vi "ABR3 Main Panel.vi"(11 "State (in)":T11) -> (3 "State":T11)   [LabVIEW 2020]
uses:
  epl-vi-lib/Utility VIs/Buttons/KCheckmarkBoolean 2.ctl
  epl-vi-lib/Utility VIs/Type Defs/Left-Right ring.ctl
  epl-vi-lib/Signal Synthesis VIs/Controls/Advanced Filter XCtl/Advanced Filter XCtl.xctl
  CFTS Main Panel SubVIs/CFTS-Experiment State.ctl
  TypeDefs/ABR3-Analysis State.ctl
  Threshold Estimation VIs/ABR3-Threshold Estimation Result.ctl
  TypeDefs/ABR3-Masker Spec.ctl
  epl-vi-lib/Signal Synthesis VIs/Controls/Level XCtl/Level XCtl.xctl
  TypeDefs/ABR3-Parameters.ctl
  TypeDefs/ABR3-Stimulus.ctl
  TypeDefs/ABR-Waveform Enum.ctl
  epl-vi-lib/Signal Synthesis VIs/Filter VIs/Filter-Bandwidth Units.ctl
  epl-vi-lib/Signal Synthesis VIs/Controls/Level XCtl/Level Units.ctl
  TypeDefs/ABR3-Sequence Spec.ctl
  TypeDefs/ABR3-Controls.ctl
  TypeDefs/ABR3-Response.ctl
  TypeDefs/ABR3-Hidden Params.ctl
  Threshold Estimation VIs/ABR3-Threshold Estimation Parameters.ctl
  <vilib>/Utility/sysdir.llb/System Directory Type.ctl
panel:
  out "Thr":string caption="Threshold (dB SPL)"
  out "User":string
  out "Run #":u16
  out "ID #":u16
  in  "Presets":u16(ring) items=["bpn", "memr chirp", "signal only", "test controls", "test", "with masker", "--- defaults ---"]
  out "resume signal":bool
  out "Masker state":bool
  in  "Last user":string
  out "exit signal":bool
  in  "Tab Control":enum32{"Stimulus", "Masker"}(tab)=enum."Masker"
  in  "Stimulus":T3={"Ear"=enum."Left", "Waveform"=enum."FILE", "Frequency (kHz)"="", "Rep rate (/sec)"=80.0, "Alternate Polarity"=FALSE, "Filenames"="", "Level (dB SPL)"=30.0, "Folder"=path "", "Chirp"={"Type"=enum."AN latency-corrected", "Duration (ms)"=30.0, "Fmin (kHz)"=30.0, "Fmax (kHz)"=80.0, "Precompensate"=FALSE}, "Noise"={"Seed"=0.0, "InvFilt"=FALSE, "Audiogram Comp"=FALSE, "Audiogram File"=path "", "Filter"={"Type"=enum."Lowpass", "CF (kHz)"=0.0, "BW (kHz)"=0.0, "Cascade"=FALSE, "Quadrature"=FALSE, "Scale Factor"=0.0, "Stages"=[], "Class"=enum."Elliptic", "Order"=0, "BWUnits"=enum."Linear"}}}
  in  "File browse":bool
  in  "Masker":T4
  out "Running":bool
  out "Abort":bool
  in  "Controls":T6
  in  "Sequence":T7={"Start (dB)"=20, "Stop (dB)"=80, "Step (dB)"=5, "Var"=enum."Signal", "Order"=enum."Sequential"} {"Start (dB)" step=5}
  in  "Response":T8={"Gain"=10000, "Averages"=512, "Window (ms)"=8.5, "Thr Fast Steps"=1.5, "AI Fs"=25000.0} {"Thr Fast Steps" format="%.2f"; "Window (ms)" format="%.2f"}
  in  "CAP or ABR":enum16{"CAP", "ABR"}(ring)=enum."ABR" caption="Measure what"
  out "CM":cluster{dbl[], dbl[]}[](graph) caption="\"CM\""
  out "Neural":cluster{dbl[], dbl[]}[](graph)
  out "load params":bool
  out "redisplay":bool
  out "settings":path
  in  "finished":errorcluster
  out "Wave 1":cluster{dbl[], dbl[]}[](graph)
  out "Analysis":T9
  out "kHz":dbl=35.0
  out "MAX SPL":dbl=113.05999755859375 format="%.2f"
  out "SPL":dbl=35.0
  out "DataPath":path
  in  "Normalize traces":T12=TRUE caption="Normalize individual traces"
  in  "Start":bool
  in  "Exit":bool
  in  "Stop":bool
  out "I-O":cluster{dbl[], dbl[]}[](graph)
  in  "NOTES":string
  # "Level"
  # "Controls"
  # "Running Average"
  # "Response"
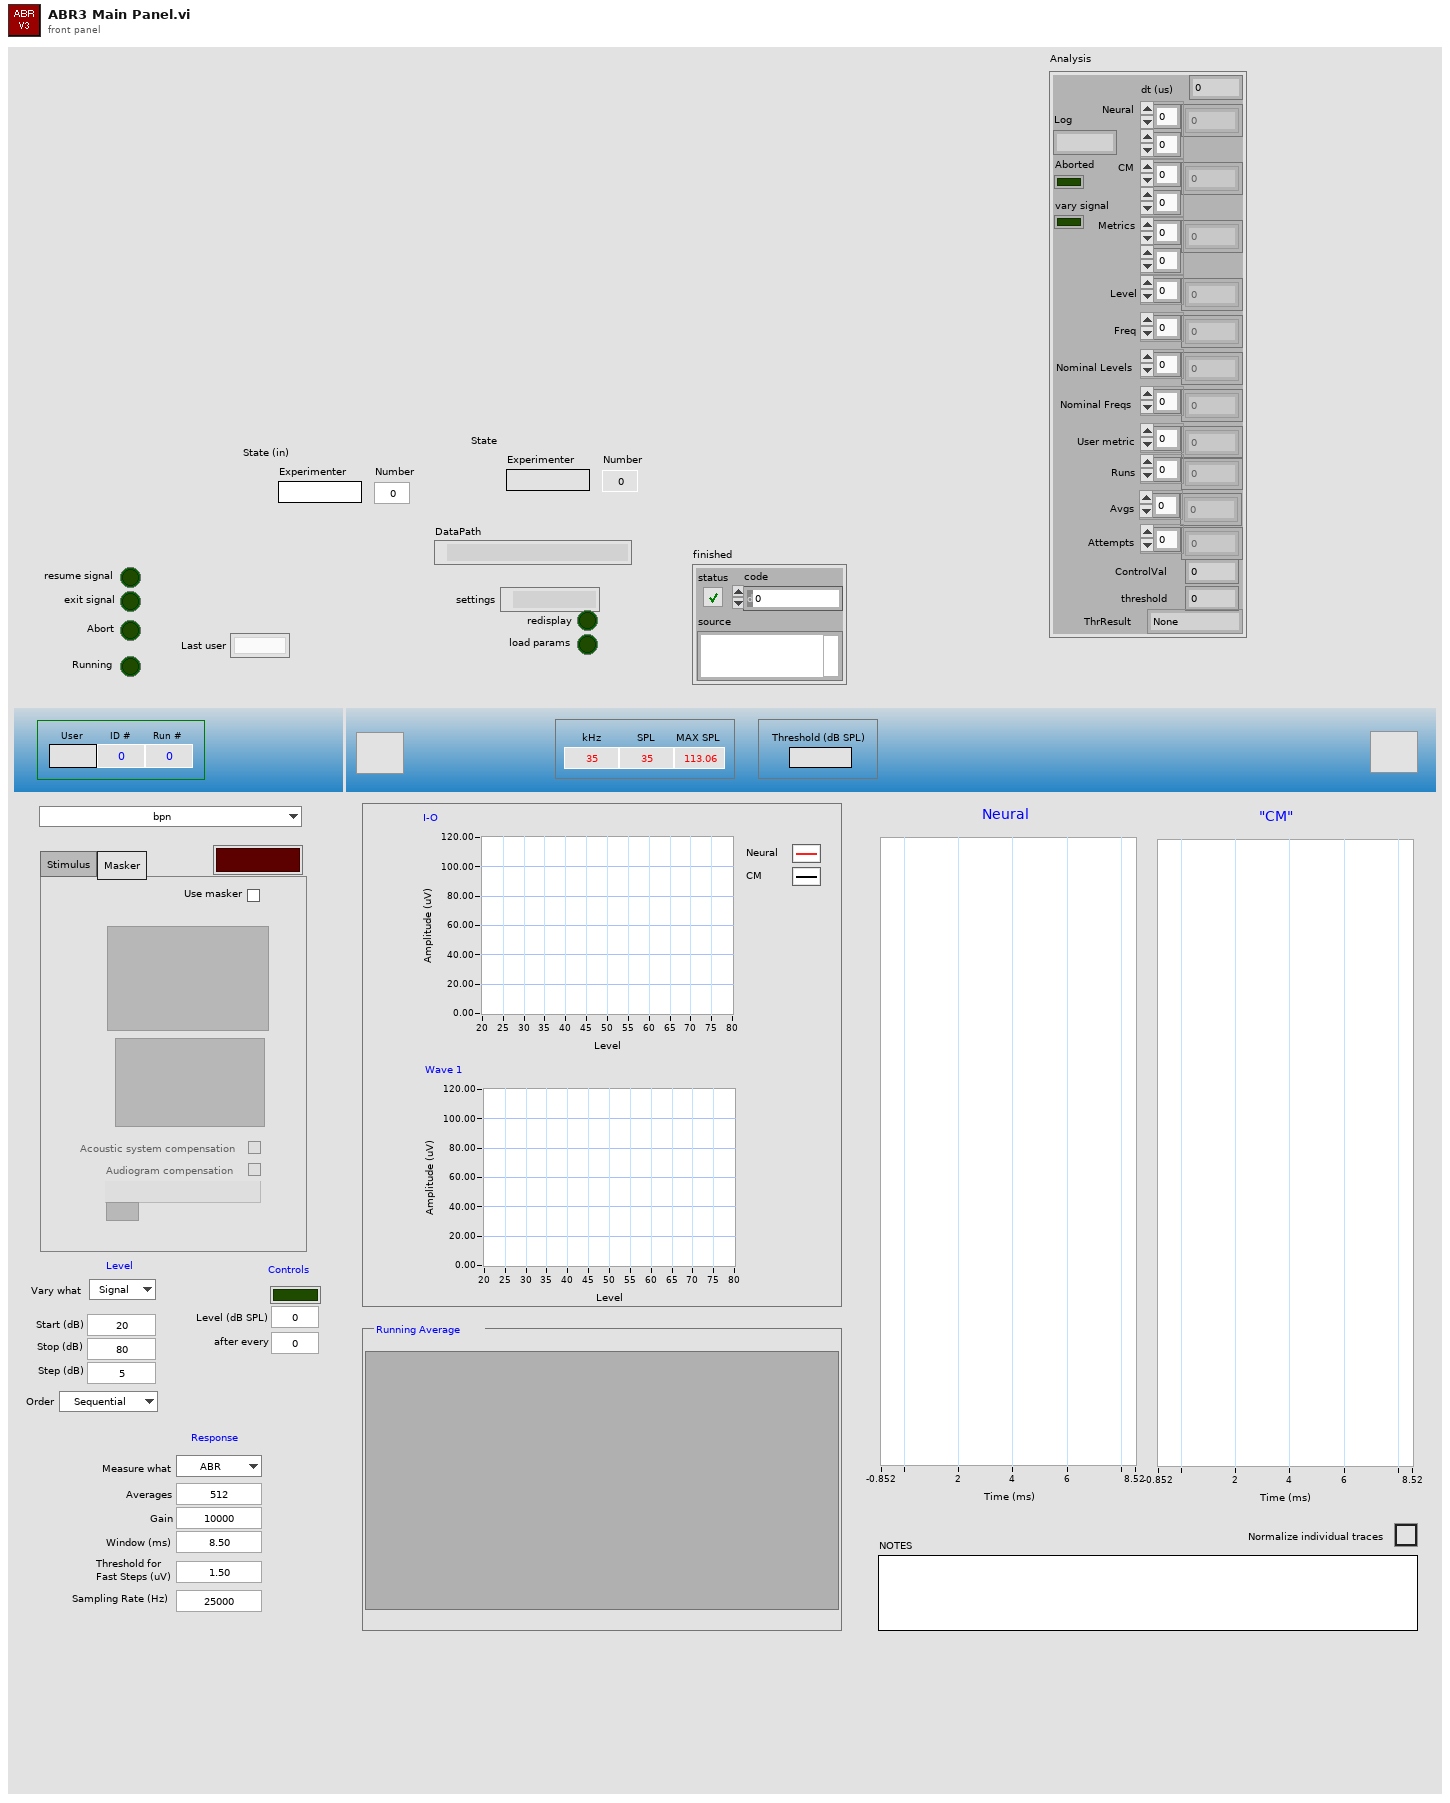
[diagram p1: front panel]
types:
  T1 = typedef "Left-Right ring.ctl" = enum16{"Right", "Left"}
  T2 = typedef "Filter-Bandwidth Units.ctl" = enum16{"Linear", "Octaves", "Min-Max"}
  T3 = cluster{"Ear":T1, "Waveform":enum16{"TONE PIP", "CLICK", "FILE", "CHIRP", "NOISE"}, "Frequency (kHz)":string, "Rep rate (/sec)":dbl, "Alternate Polarity":bool, "Filenames":string, "Level (dB SPL)":dbl, "Folder":path, "Chirp":cluster{"Type":enum16{"AN latency-corrected", "Arbitrary"}, "Duration (ms)":dbl, "Fmin (kHz)":dbl, "Fmax (kHz)":dbl, "Precompensate":bool}, "Noise":cluster{"Seed":dbl, "InvFilt":bool, "Audiogram Comp":bool, "Audiogram File":path, "Filter":cluster{"Type":enum16{"Lowpass", "Highpass", "Bandpass", "Bandstop", "OFF"}, "CF (kHz)":dbl, "BW (kHz)":dbl, "Cascade":bool, "Quadrature":bool, "Scale Factor":dbl, "Stages":cluster{"IIR Filter":cluster{"filter structure":enum32{"IIR 2nd Order", "IIR 4th Order"}, "Reverse Coefficients":dbl[], "Forward Coefficients":dbl[]}, "State":dbl[]}[], "Class":enum16{"Elliptic", "Butterworth"}, "Order":i32, "BWUnits":T2}}}
  T4 = typedef "ABR3-Masker Spec.ctl" = cluster{"Filter":cluster{"Type":enum16{"Lowpass", "Highpass", "Bandpass", "Bandstop", "OFF"}, "CF (kHz)":dbl, "BW (kHz)":dbl, "Cascade":bool, "Quadrature":bool, "Scale Factor":dbl, "Stages":cluster{"IIR Filter":cluster{"filter structure":enum32{"IIR 2nd Order", "IIR 4th Order"}, "Reverse Coefficients":dbl[], "Forward Coefficients":dbl[]}, "State":dbl[]}[], "Class":enum16{"Elliptic", "Butterworth"}, "Order":i32, "BWUnits":T2}, "Use masker":bool, "Level":cluster{"Level":dbl, "Units":T5, "Max":dbl, "Multiplier":dbl, "Cal File":path, "Cal":cluster{"Freq (Hz)":dbl[], "Mag (dB SPL)":dbl[], "Phase (deg)":dbl[]}}, "Audiogram Comp":bool, "Audiogram File":path, "InvFilt":bool}
  T5 = typedef "Level Units.ctl" = enum16{"dB atten", "dB SPL", "dB re 1 Vrms", "dB V/Hz½", "mW", "dB HL", "Volts", "dB mW"}
  T6 = cluster{"on":bool, "Dur (ms)":dbl, "spacing":i32}
  T7 = cluster{"Start (dB)":i32, "Stop (dB)":i32, "Step (dB)":i32, "Var":enum16{"Signal", "Masker"}, "Order":enum16{"Sequential", "Random"}}
  T8 = cluster{"Gain":i32, "Averages":i32, "Window (ms)":sgl, "Thr Fast Steps":sgl, "AI Fs":dbl}
  T9 = typedef "ABR3-Analysis State.ctl" = cluster{"dt (us)":dbl, "Neural":dbl[][], "CM":dbl[][], "Metrics":dbl[][], "Level":dbl[], "Freq":dbl[], "Nominal Levels":dbl[], "Nominal Freqs":dbl[], "User metric":dbl[], "Runs":i32[], "Avgs":i32[], "Attempts":i32[], "Log":string, "Aborted":bool, "ControlVal":dbl, "threshold":dbl, "vary signal":bool, "ThrResult":T10}
  T10 = typedef "ABR3-Threshold Estimation Result.ctl" = enum16{"None", "Power", "Sigmoid", "Power (noisy)", "Suprathreshold", "Invalid"}
  T11 = typedef "CFTS-Experiment State.ctl" = cluster{"Experimenter":string, "Number":u32, "Right":string, "Left":string, "Data Folder":path, "State File":path, "Version Info":string, "End Exposure Time":dbl, "Exposure Duration":string, "Run #":cluster{"CAP":i16, "ABR":i16, "DP":i16, "VsEP":i16, "MeasSeq":i16, "SubSeq":i16, "SFOAE":i16}}
  T12 = typedef "KCheckmarkBoolean 2.ctl" = bool
  T13 = typedef "ABR3-Threshold Estimation Parameters.ctl" = cluster{"Tmin (ms)":dbl, "Tmax (ms)":dbl, "CC criterion":dbl, "adjR2 criterion":dbl}
  T14 = typedef "ABR3-Parameters.ctl" = cluster{"CAP or ABR":enum16{"CAP", "ABR"}, "Stimulus":T15, "Masker":T4, "Sequence":T17, "Controls":T18, "Response":T19, "Hidden":T20}
  T15 = typedef "ABR3-Stimulus.ctl" = cluster{"Ear":T1, "Waveform":T16, "Frequency (kHz)":string, "Rep rate (/sec)":dbl, "Alternate Polarity":bool, "WavFiles":string, "Level (dB SPL)":dbl, "WavFolder":path, "Chirp":cluster{"Type":enum16{"AN latency-corrected", "Arbitrary"}, "Duration (ms)":dbl, "Fmin (kHz)":dbl, "Fmax (kHz)":dbl, "precompensate":bool}, "Noise":cluster{"Seed":i32, "InvFilt":bool, "AWeight":bool, "afile":path, "Filter":cluster{"Type":enum16{"Lowpass", "Highpass", "Bandpass", "Bandstop", "OFF"}, "CF (kHz)":dbl, "BW (kHz)":dbl, "Cascade":bool, "Quadrature":bool, "Scale Factor":dbl, "Stages":cluster{"IIR Filter":cluster{"filter structure":enum32{"IIR 2nd Order", "IIR 4th Order"}, "Reverse Coefficients":dbl[], "Forward Coefficients":dbl[]}, "State":dbl[]}[], "Class":enum16{"Elliptic", "Butterworth"}, "Order":i32, "BWUnits":T2}}}
  T16 = typedef "ABR-Waveform Enum.ctl" = enum16{"TONE PIP", "CLICK", "FILE", "CHIRP", "NOISE", "VERHULST"}
  T17 = typedef "ABR3-Sequence Spec.ctl" = cluster{"Start (dB)":i32, "Stop (dB)":i32, "Step (dB)":i32, "Var":enum16{"Signal", "Masker"}, "Order":enum16{"Sequential", "Random"}}
  T18 = typedef "ABR3-Controls.ctl" = cluster{"on":bool, "value":dbl, "spacing":i32}
  T19 = typedef "ABR3-Response.ctl" = cluster{"Gain":i32, "Averages":i32, "Window (ms)":sgl, "Thr Fast Steps":sgl, "AI Fs":dbl}
  T20 = typedef "ABR3-Hidden Params.ctl" = cluster{"AO Samp Rate Hz":dbl, "Duration (ms)":dbl, "Ramp (ms)":dbl, "Click width (us)":dbl}
  T21 = cluster{"Params":T14, "Threshold Estimation":T13}
  T22 = cluster{"I-O":refnum<vi>, "Neural":refnum<vi>, "CM":refnum<vi>, "Wave 1":refnum<vi>}
  T23 = typedef "ABR3-Runtime Data.ctl" = cluster{"Ceiling":dbl, "Threshold":dbl, "Crossed?":bool, "Step":i32, "Stop":i32, "Avgs":i32, "Level":dbl, "AI Npts":i32, "Doubled?":bool, "Gain":dbl, "NWindowPts":i32, "dt":dbl, "Cal":path, "Freq":dbl, "AO Channels":i32[], "AltPol":bool, "AO Npts":i32, "AO Fs":dbl, "Start":i32, "Stop max":i32, "Ear":T1, "Waveform":T16, "RepRate":dbl, "CAP or ABR":u16, "LMasker":dbl, "SeqVar":T24, "Reps/buffer":i32, "Avg Mode":enum16{"Neural/CM", "ANOW"}, "Wav":path, "Order":enum16{"Sequential", "Random"}, "Levels":dbl[], "ControlVal":dbl, "innerIndex":i32, "indexStep":i32}
  T24 = typedef "ABR3-Seq Var Enum.ctl" = enum16{"Signal Level", "Masker Level"}
  T25 = typedef "Stimulus Channel (Full).xctl/Full Stimulus Channel Data.ctl" = cluster{"Waveform":T26, "Filter":T43, "Burst":T44, "Level":T45, "Name":string, "Advanced":T46, "SAM":T47}
  T26 = typedef "Waveform XCtl.xctl/Waveform Data.ctl" = cluster{"Type":T27, "Tone":T28, "Pulse Train":T29, "Noise":T32, "File":T33, "FMSweep":T34, "Chirp Train":T35, "Complex Tone":cluster{"Params":T37, "Data":T39}, "Moving Ripple":T40}
  T27 = typedef "Waveform Enum.ctl" = enum16{"OFF", "Tone", "Noise", "Pulse Train", "File", "FM Sweep", "Chirp Train", "Complex Tone", "FM Tone", "Moving Ripple"}
  T28 = typedef "Tone Params.ctl" = cluster{"Frequency (kHz)":dbl, "Last Freq":dbl, "Last Phase":dbl}
  T29 = typedef "Pulse Train Params.ctl" = cluster{"Pulse width (us)":dbl, "Pulse rate (Hz)":dbl, "Gap (ms)":dbl, "Polarity":T30, "PT State":T31, "Asynch":bool}
  T30 = typedef "Pulse Polarity.ctl" = enum16{"POS", "NEG", "POS-NEG", "NEG-POS"}
  T31 = typedef "PT-Continuous State.ctl" = cluster{"Template":dbl[], "Nperiod":i32, "Index":i32, "Pulse Rate (Hz)":dbl, "Phase (cycles)":dbl, "Noff":i32}
  T32 = typedef "Noise Params.ctl" = cluster{"InvFilt":bool, "Noise":dbl[], "CurPt":i32, "Aweight":bool, "Seed":i32, "afile":path}
  T33 = typedef "StimFile-Params.ctl" = cluster{"Filename":path, "Signal":dbl[], "Channel":i32, "stream":bool, "offset":i32, "nreps":i32, "loops":i32, "Randomize":bool, "order":i32[], "Seed":i32, "Tokens":i32}
  T34 = typedef "FM Sweep Params.ctl" = cluster{"Rate (oct/s)":dbl, "Fmin (Hz)":dbl, "Fmax (Hz)":dbl, "Ramp (ms)":dbl, "Linear":bool}
  T35 = typedef "Chirp Train.ctl" = cluster{"Params":T36, "Data":cluster{"WF":dbl[]}}
  T36 = typedef "Chirp Train Params.ctl" = cluster{"Fmin (kHz)":dbl, "Fmax (kHz)":dbl, "Compensate":bool, "Duration (ms)":dbl}
  T37 = typedef "CT-Params.ctl" = cluster{"F0 (Hz)":dbl, "Band":cluster{"Flow (Hz)":dbl, "Fhigh (Hz)":dbl}, "Phase":T38, "Min F0 (Hz)":dbl, "Max F0 (Hz)":dbl, "ContinRandPhase":bool, "Max peak factor":dbl, "Max mod depth":dbl, "MinHarmNum":i32, "MaxHarmNum":i32, "Level Mode":enum16{"per component", "overall rms"}, "% jitter":dbl}
  T38 = typedef "CT-Phase Enum.ctl" = enum16{"Cosine", "Random", "Alternating"}
  T39 = typedef "CT-Runtime Data.ctl" = cluster{"Ncomp":i32, "MinHarm":i32, "Phase":dbl[], "Amplitude":dbl[], "Npts/frame":i32, "Last F0":dbl, "Fmin":dbl, "Fmax":dbl, "Lslope":dbl, "randphase":bool, "overall rms":bool, "fmult":dbl[], "jittered":bool}
  T40 = typedef "Moving Ripple.ctl" = cluster{"Params":T41, "Data":T42}
  T41 = typedef "Moving Ripple.Params.ctl" = cluster{"Fmin":dbl, "Fmax":dbl, "Density":dbl, "Velocity":dbl, "Depth":dbl, "Phase":dbl, "Comp/oct":i32}
  T42 = typedef "Moving Ripple.Data.ctl" = cluster{"Freq":dbl[], "A":dbl[], "phase":dbl[], "Phase":dbl}
  T43 = typedef "Advanced Filter XCtl.xctl/Filter Data.ctl" = cluster{"Type":enum16{"Lowpass", "Highpass", "Bandpass", "Bandstop", "OFF"}, "CF (kHz)":dbl, "BW (kHz)":dbl, "Cascade":bool, "Quadrature":bool, "Scale Factor":dbl, "Stages":cluster{"IIR Filter":cluster{"filter structure":enum32{"IIR 2nd Order", "IIR 4th Order"}, "Reverse Coefficients":dbl[], "Forward Coefficients":dbl[]}, "State":dbl[]}[], "Class":enum16{"Elliptic", "Butterworth"}, "Order":i32, "BWUnits":T2}
  T44 = typedef "Burst Control.xctl/Burst Data.ctl" = cluster{"Active":bool, "Delay (ms)":dbl, "Duration (ms)":dbl, "Ramp (ms)":dbl, "Rate (Hz)":dbl, "Trepeat (ms)":dbl, "Repeat":bool}
  T45 = typedef "Level XCtl.xctl/Level Data.ctl" = cluster{"Level":dbl, "Units":T5, "Max":dbl, "Multiplier":dbl, "Cal File":path, "Cal":cluster{"Freq (Hz)":dbl[], "Mag (dB SPL)":dbl[], "Phase (deg)":dbl[]}}
  T46 = typedef "Advanced Stimulus Options.xctl/Advanced Stimulus Options.ctl" = cluster{"Rep Mask":string, "AltPol":bool, "Var":string, "Expr":string, "Persist":bool}
  T47 = typedef "SAM Params.ctl" = cluster{"Active":bool, "Frequency (Hz)":dbl, "Depth":dbl, "Init Phase (cycles)":dbl, "phase (degrees)":dbl, "Asynch":bool}
  T48 = typedef "Multichannel (Full).xctl/Data.ctl" = T25[]
  T49 = enum8{"Enabled", "Disabled", "Disabled and Grayed Out"}
  T50 = cluster{"Shift":bool, "Ctrl":bool, "Alt":bool, "Cmd":bool, "Opt":bool}
  T51 = typedef "ABR3-Threshold Estimation Work.ctl" = cluster{"Threshold":dbl, "Criterion":dbl, "graphs":cluster{"X":dbl[], "Y":dbl[]}[], "Power2":string, "Sigmoid":string, "Result":T10}
  T52 = enum16{"TONE PIP", "CLICK", "FILE", "CHIRP", "NOISE"}
  T53 = cluster{"Params":T14, "Threshold Estimation Out":T13}
  T54 = typedef "System Directory Type.ctl" = i32
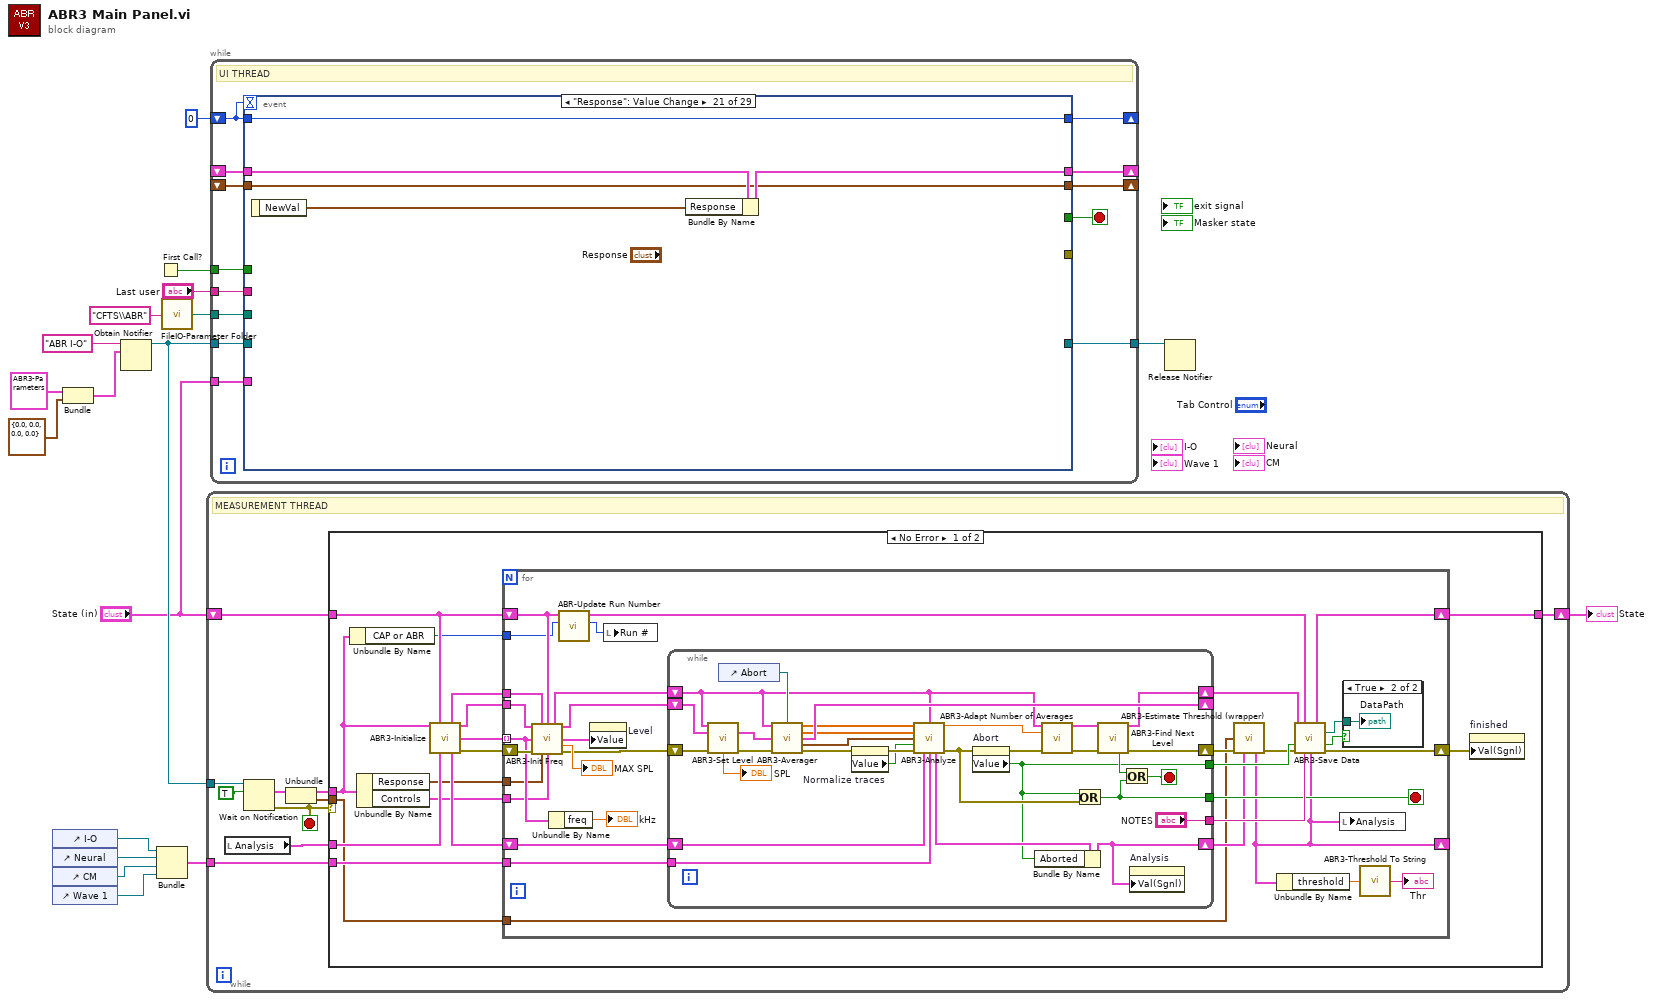
[diagram p0: block diagram]
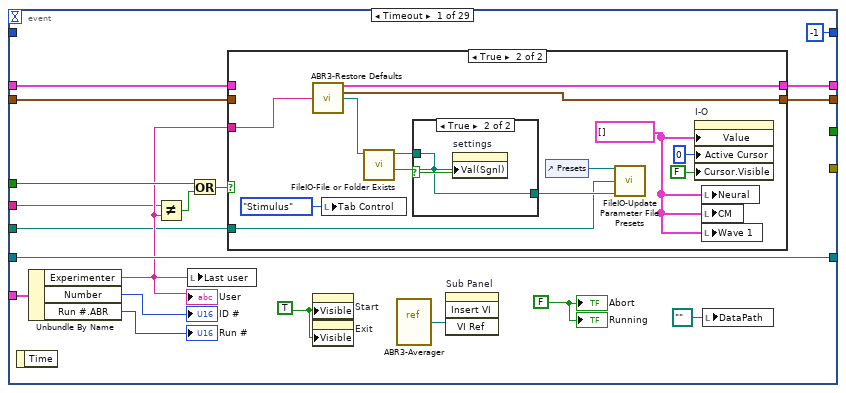
[diagram p4: hidden frame]
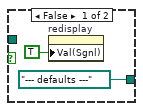
[diagram p6: hidden frame]
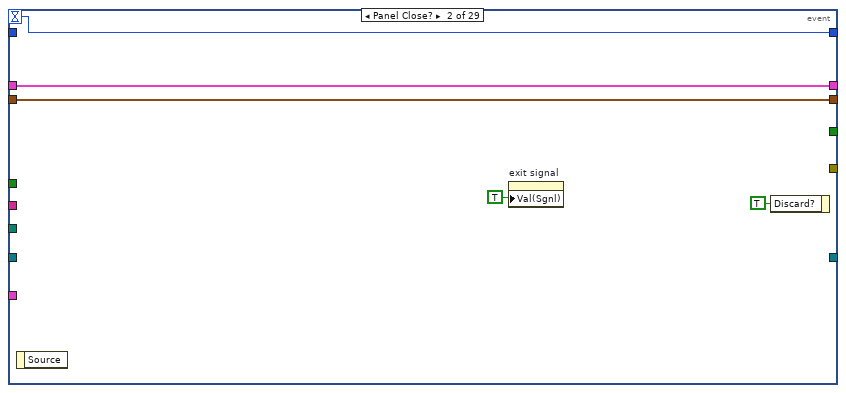
[diagram p7: hidden frame]
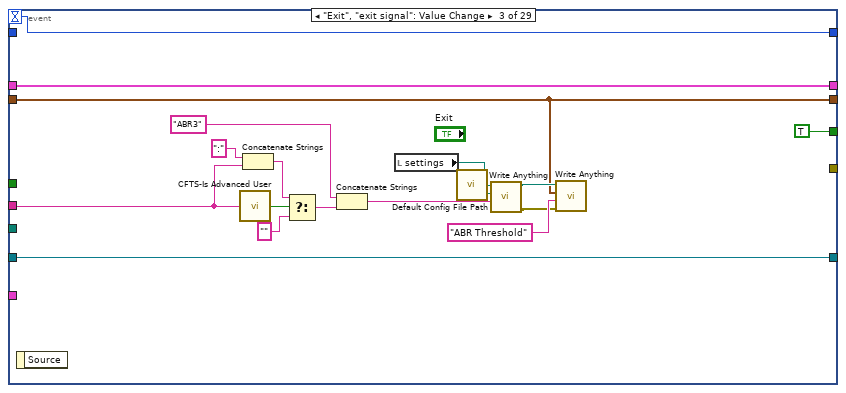
[diagram p8: hidden frame]
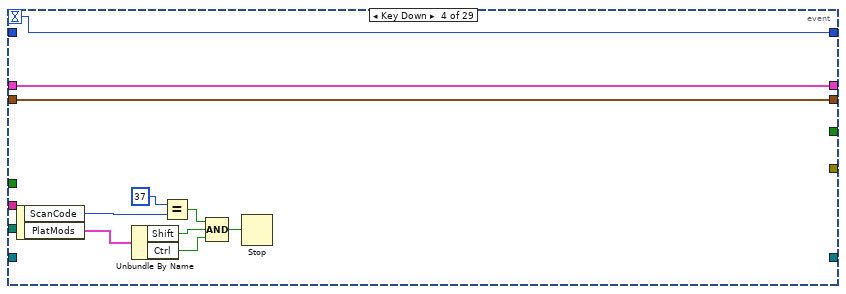
[diagram p9: hidden frame]
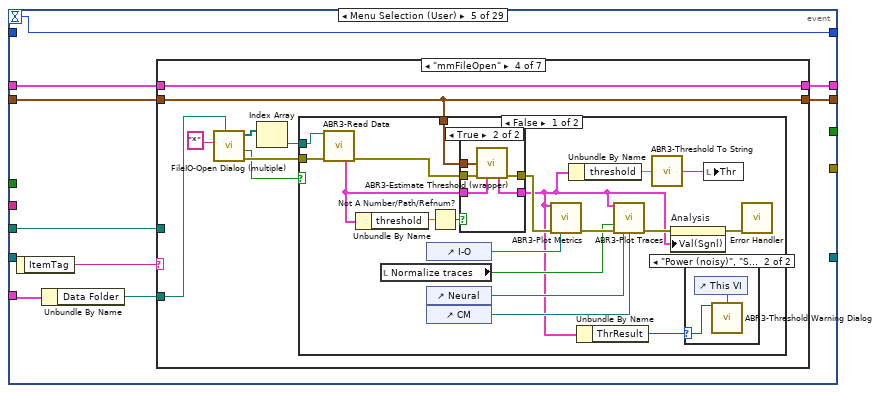
[diagram p10: hidden frame]
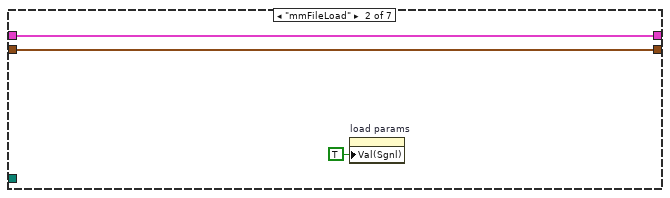
[diagram p12: hidden frame]
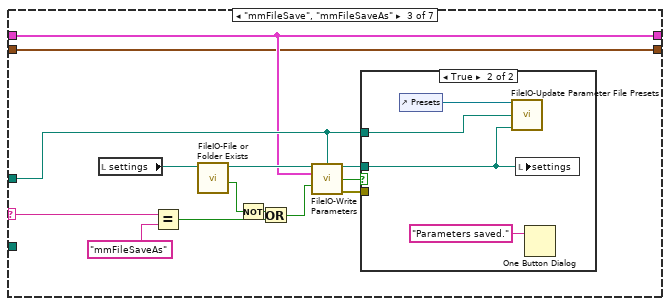
[diagram p13: hidden frame]
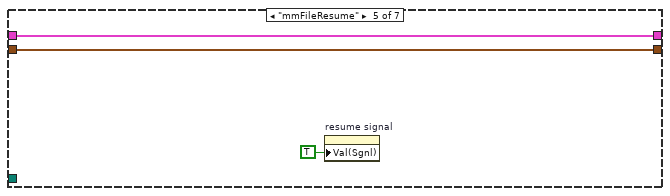
[diagram p18: hidden frame]
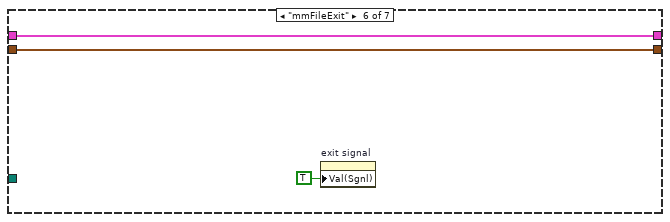
[diagram p19: hidden frame]
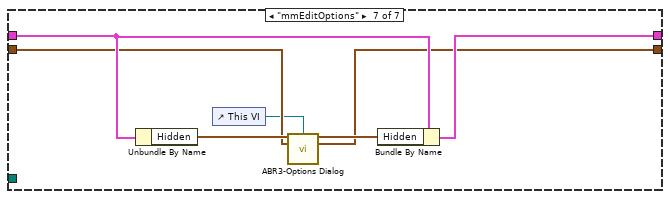
[diagram p20: hidden frame]
diagram:
  n1 = control-ref of="I-O"() -> (w9:refnum<vi>)
  n2 = control-ref of="Neural"() -> (w5:refnum<vi>)
  n3 = control-ref of="CM"() -> (w4:refnum<vi>)
  n4 = control-ref of="Wave 1"() -> (w10:refnum<vi>)
  n5 = Bundle("Params"=T14 {"CAP or ABR"=enum."ABR", "Stimulus"={"Ear"=enum."Left", "Waveform"=enum."TONE PIP", "Frequency (kHz)"="", "Rep rate (/sec)"=30.0, "Alternate Polarity"=FALSE, "WavFiles"="", "Level (dB SPL)"=30.0, "WavFolder"=path "", "Chirp"={"Type"=enum."AN latency-corrected", "Duration (ms)"=0.0, "Fmin (kHz)"=0.0, "Fmax (kHz)"=0.0, "precompensate"=FALSE}, "Noise"={"Seed"=0, "InvFilt"=FALSE, "AWeight"=FALSE, "afile"=path "", "Filter"={"Type"=enum."Lowpass", "CF (kHz)"=0.0, "BW (kHz)"=0.0, "Cascade"=FALSE, "Quadrature"=FALSE, "Scale Factor"=0.0, "Stages"=[], "Class"=enum."Elliptic", "Order"=0, "BWUnits"=enum."Linear"}}}, "Masker"={"Filter"={"Type"=enum."Lowpass", "CF (kHz)"=0.0, "BW (kHz)"=0.0, "Cascade"=FALSE, "Quadrature"=FALSE, "Scale Factor"=0.0, "Stages"=[], "Class"=enum."Elliptic", "Order"=0, "BWUnits"=enum."Linear"}, "Use masker"=FALSE, "Level"={"Level"=0.0, "Units"=enum."dB atten", "Max"=0.0, "Multiplier"=0.0, "Cal File"=path "", "Cal"={"Freq (Hz)"=[], "Mag (dB SPL)"=[], "Phase (deg)"=[]}}, "Audiogram Comp"=FALSE, "Audiogram File"=path "", "InvFilt"=FALSE}, "Sequence"={"Start (dB)"=20, "Stop (dB)"=80, "Step (dB)"=5, "Var"=enum."Signal", "Order"=enum."Sequential"}, "Controls"={"on"=FALSE, "value"=0.0, "spacing"=0}, "Response"={"Gain"=10000, "Averages"=512, "Window (ms)"=8.5, "Thr Fast Steps"=8.5, "AI Fs"=0.0}, "Hidden"={"AO Samp Rate Hz"=100000.0, "Duration (ms)"=5.0, "Ramp (ms)"=0.5, "Click width (us)"=0.0}}, "Threshold Estimation"=T13 {"Tmin (ms)"=0.0, "Tmax (ms)"=0.0, "CC criterion"=0.0, "adjR2 criterion"=0.0}) -> (w1:T21)  [unwired: 1 in]
  n6 = Obtain Notifier(name (unnamed)="ABR I-O", notification data type=w1) -> (notifier out=w17:refnum<notifier>)  [unwired: 2 in, 2 out]
  n7 = First Call?() -> (First Call?: T/F=w14:bool)
  n8 = Bundle("I-O"=w9, "Neural"=w5, "CM"=w4, "Wave 1"=w10) -> (w8:T22)  [unwired: 1 in]
  n9 = call "FileIO-Parameter Folder.vi"("subfolder"="CFTS\\ABR" ("name or relative path")) -> ("parameter folder"=w6:path)  [unwired: 4 in]
  n10 = while {
    tunnel: w17 -> [w27]
    shift-right: [w24] -> w12
    shift-left: "State (in)" -> [w25]
    tunnel: w8 -> [w23]
    stop <- w26 stop-if-true
    # "MEASUREMENT THREAD"
    n11 = local read "Analysis"() -> (w21:T9)
    n12 = Wait on Notification(notifier=w27, ignore previous (F)=TRUE) -> (notification=w22:T21, error out=w26:errorcluster)  [unwired: 2 in, 2 out]
    n13 = Unbundle(w22) -> ("Params"=w20:T14, "Threshold Estimation"=w19:T13)
    n14 = case shown="No Error" w26 {
      tunnel: w25 -> [w39 w108]
      tunnel: [w38 w108] -> w24
      tunnel: w23 -> [w37 _]
      tunnel: w20 -> [w33 _]
      tunnel: w21 -> [w35 _]
      tunnel: w19 -> [w29 _]
      frame No Error {
        n15 = Unbundle By Name(w33) -> ("CAP or ABR"=w30:enum16{"CAP", "ABR"})
        n16 = Unbundle By Name(w33) -> ("Response"=w32:T19, "Controls"=w31:T18)
        n17 = call "ABR3-Initialize.vi"("Params"=w33, "State"=w39, "Analysis In"=w35) -> ("Runtime"=w42:T23, "Stimulus out"=w40:T25[], "outerVals"=w34:cluster{"wavfile":path, "freq":dbl}[], "Analysis"=w41:T9, "error out"=w43:errorcluster)  [unwired: 8 in]
        n18 = for {
          tunnel: w42 -> [w75]
          tunnel: w40 -> [w69]
          tunnel: w37 -> [w72]
          shift-right: [w45] -> _
          shift-left: w41 -> [w59]
          shift-right: [w67] -> w38
          shift-left: w39 -> [w58]
          shift-right: [w68] -> w36
          shift-left: w43 -> [w76]
          tunnel: w34 -> [w55] mode=indexing
          tunnel: w32 -> [w53]
          tunnel: w31 -> [w52]
          tunnel: w30 -> [w51]
          tunnel: w29 -> [w44]
          stop <- w61 stop-if-true
          n19 = call "ABR3-Init Freq.vi"("StimChans"=w69, "Runtime"=w75, "State (in)"=w58, "outerVal"=w55, "error in (no error)"=w76, "Response"=w53, "Controls"=w52) -> ("Runtime out"=w74:T23, "Stimulus (out)"=w70:T25[], "Masker Level"=w60:T45, "Ceiling"=→"MAX SPL":dbl, "error out"=w71:errorcluster)  [unwired: 4 in]
          n20 = Unbundle By Name(w55) -> ("freq"=→"kHz":dbl)
          n21 = call "ABR-Update Run Number.vi"("CAP or ABR"=w51, "State (in)"=w58) -> ("run #"=w56:i16, "State (out)"=w57:T11)  [unwired: 7 in, 1 out]
          n22 = property on="Level" class="Level XCtl (strict)"("Value"=w60) -> ()  [unwired: 2 in, 2 out]
          n23 = local write "Run #"(w56) -> ()
          n24 = while {
            shift-right: [w100] -> w65
            shift-left: w74 -> [w79]
            shift-right: [w84] -> w48
            shift-left: w59 -> [w95]
            tunnel: w72 -> [w77]
            tunnel: [w83] -> w62
            shift-right: [w106] -> _
            shift-left: w70 -> [w94]
            tunnel: ["NOTES"] -> w64
            tunnel: [w91] -> w61
            shift-right: [w103] -> w50
            shift-left: w71 -> [w101]
            stop <- w105 stop-if-true
            # "5. Stop DAQ"
            # "stepsize"
            # "max SPL"
            # "array of levels"
            # "current SPL"
            n25 = call "ABR3-Set Level.vi"("Runtime"=w79, "StimChans"=w94, "error in (no error)"=w101) -> ("StimChans out"=w93:T25[], "Level"=→"SPL":dbl, "error out"=w90:errorcluster)  [unwired: 10 in]
            n26 = control-ref of="Abort"() -> (w104:refnum<vi>)
            n27 = call "ABR3-Averager.vi"("Runtime"=w79, "Abort"=w104, "StimChans"=w93, "error in (no error)"=w90) -> ("Neural (uV)"=w99:dbl[], "microphonic (uV)"=w98:dbl[], "StimChans out"=w106:T48, "Averaging data"=w85:cluster{i32, i32}, "error out"=w89:errorcluster)  [unwired: 7 in]
            n28 = property on="Normalize traces" class="Bool (strict)"(error in=w89) -> (error out=w97:errorcluster, "Value"=w86:T12)  [unwired: 1 in, 1 out]
            n29 = call "ABR3-Analyze.vi"("Neural (uV)"=w99, "Runtime"=w79, "microphonic (uV)"=w98, "Averaging data"=w85, "Normalize individual?"=w86, "error in"=w97, "Analysis"=w95, "Graphs"=w77) -> ("spread value"=w80:dbl, "Analysis out"=w88:T9, "error out"=w87:errorcluster)  [unwired: 5 in]
            n30 = property on="Abort" class="Bool (strict)"(error in=w87) -> (error out=w81:errorcluster, "Value"=w83:bool)  [unwired: 1 in, 1 out]
            n31 = Bundle By Name(cluster=w88, "Aborted"=w83) -> (w84:T9)
            n32 = call "ABR3-Adapt Number of Averages.vi"("Runtime"=w79, "Amplitude"=w80, "error in (no error)"=w81) -> ("Runtime out"=w78:T23, "error out"=w82:errorcluster)  [unwired: 11 in]
            n33 = Or(x=w83, y=w87) -> (x .or. y?=w91:bool)
            n34 = call "ABR3-Find Next Level.vi"("Runtime"=w78, "error in (no error)"=w82) -> ("Runtime out"=w100:T23, "Finished"=w102:bool, "error out"=w103:errorcluster)  [unwired: 11 in]
            n35 = Or(x=w102, y=w91) -> (x .or. y?=w105:bool)
            n36 = property on="Analysis" class="Clust (strict)"("Val(Sgnl)"=w84) -> ()  [unwired: 2 in, 2 out]
          }
          n37 = call "ABR3-Estimate Threshold (wrapper).vi"("Threshold Estimation"=w44, "error in (no error)"=w50, "Analysis (in)"=w48) -> ("Analysis (out)"=w45:T9, "error out"=w49:errorcluster)  [unwired: 10 in, 1 out]
          n38 = Unbundle By Name(w45) -> ("threshold"=w47:dbl)
          n39 = call "ABR3-Save Data.vi"("Runtime"=w65, "State (in)"=w57, "Aborted?"=w62, "error in (no error)"=w49, "Notes"=w64, "Analysis"=w45) -> ("State (out)"=w67:T11, "Datafile path"=w66:path, "Saved?"=w63:bool, "error out"=w68:errorcluster)  [unwired: 5 in, 1 out]
          n40 = local write "Analysis"(w45) -> ()
          n41 = case shown="True" w63 {
            tunnel: w66 -> [_ w107]
            frame False {
            }
            frame True {
              "DataPath" <- w107
            }
          }
          n42 = call "ABR3-Threshold To String.vi"("Threshold"=w47) -> ("String"=→"Thr":string)
        }
        n43 = property on="finished" class="Clust (strict)"("Val(Sgnl)"=w36) -> ()  [unwired: 2 in, 2 out]
      }
      frame Error {
      }
    }
  }
  "State" <- w12
  n44 = while {
    tunnel: w17 -> [w120]
    tunnel: [w119] -> w18
    shift-right: [w118] -> _
    shift-left: 0 -> [w114]
    tunnel: w14 -> [w117]
    tunnel: "State (in)" -> [w116]
    tunnel: "Last user" -> [w115]
    shift-right: [w112] -> _
    shift-left: _ -> [w113]
    tunnel: w6 -> [w111]
    shift-right: [w110] -> _
    shift-left: _ -> [w109]
    stop <- w121 stop-if-true
    # "UI THREAD"
    n45 = event shown="[20] \"Response\": Value Change" {
      selector: _ -> [_ _ _ _ _ _ _ _ _ _ _ _ _ _ _ _ _ _ _ _ _ _ _ _ _ _ _ _ _]
      dyn-events: _ -> [_ _ _ _ _ _ _ _ _ _ _ _ _ _ _ _ _ _ _ _ _ _ _ _ _ _ _ _ _]
      timeout: w114 -> [_ w163 w179 w184 w200 _ _ _ _ _ _ _ _ _ w378 _ _ w419 _ _ _ w446 w457 w472 _ w503 w513 w521 w545]
      tunnel: [_ _ TRUE _ _ _ _ _ _ _ _ _ _ _ _ _ _ _ _ _ _ _ _ _ _ _ _ _ _] -> w121
      tunnel: w120 -> [w134 _ w180 _ _ _ _ _ _ _ _ _ _ _ _ _ _ _ _ _ _ w441 w454 _ _ _ _ _ _]
      tunnel: [w134 _ w180 _ _ _ _ _ _ _ _ _ _ _ _ _ _ _ _ _ _ _ _ _ _ _ _ _ _] -> w119
      tunnel: [-1 w163 w179 w184 w200 w278 w283 w295 w303 w314 w320 w352 w364 w369 w378 w406 w411 w419 w427 w432 w437 w446 w457 w472 w486 w503 w513 w521 w545] -> w118
      tunnel: w117 -> [w131 _ _ _ _ _ _ _ _ _ _ _ _ _ _ _ _ _ _ _ _ _ _ _ _ _ _ _ _]
      tunnel: w116 -> [w132 _ _ _ w199 _ _ _ _ _ _ _ _ _ _ _ _ _ _ _ _ _ _ _ _ _ _ _ _]
      tunnel: w115 -> [w127 _ w168 _ _ _ _ _ _ _ _ _ _ _ _ _ _ _ _ _ _ _ _ _ _ _ _ _ _]
      tunnel: [_ _ _ _ _ _ _ _ _ _ _ _ _ _ _ _ _ _ _ _ _ _ _ _ _ w493 _ _ _] -> _
      tunnel: w114 -> [_ _ _ _ _ w278 w283 w295 w303 w314 w320 w352 w364 w369 _ w406 w411 _ w427 w432 w437 _ _ _ w486 _ _ _ _]
      tunnel: w113 -> [w126 w160 w178 w183 w195 w277 w282 w294 w298 w313 w318 w343 w363 w368 w373 w405 w410 w413 w426 w431 w436 w440 w453 w471 w482 w492 w511 w520 w538]
      tunnel: [w125 w160 w178 w183 w194 w277 w282 w294 w297 w313 w318 w340 w362 w367 w373 w405 w409 w413 w425 w430 w435 w440 w453 w471 w482 w491 w511 w520 w538] -> w112
      tunnel: w111 -> [w124 _ _ _ w196 _ _ _ w300 _ w317 w341 _ _ _ _ _ _ _ _ _ _ _ _ _ _ _ _ _]
      tunnel: [w123 w159 w164 w182 w192 w273 w279 w284 w296 w308 w315 w339 w360 w365 w370 w401 w407 w412 w423 w428 w433 w439 w452 w470 w476 w489 w510 w519 w536] -> w110
      tunnel: w109 -> [w122 w159 w164 w182 w193 w273 w279 w284 w296 w308 w315 w339 w360 w365 w370 w401 w407 w412 w423 w428 w433 w439 w452 w470 w476 w489 w510 w519 w536]
      event Timeout {
        w136 = FALSE ("quitting")
        w137 = TRUE
        n46 = event-data() -> ()  [unwired: 1 in, 1 out]
        n47 = Unbundle By Name(w132) -> ("Experimenter"=w128:string, "Number"=→"ID #":u32, "Run #.ABR"=→"Run #":i16)
        "User" <- w128
        n48 = Not Equal?(x=w127, y=w128) -> (x != y?=w129:bool)
        n49 = local write "Last user"(w128) -> ()
        n50 = Or(x=w131, y=w129) -> (x .or. y?=w130:bool)
        n51 = case shown="True" w130 {
          tunnel: w128 -> [_ w149]
          tunnel: w126 -> [w142 _]
          tunnel: [w142 w155] -> w125
          tunnel: w124 -> [_ w148]
          tunnel: [w141 w143] -> w123
          tunnel: w122 -> [w141 _]
          frame False {
          }
          frame True {
            w146 = cluster{dbl[], dbl[]}[] [] ("TONE I-O")
            n52 = call "ABR3-Restore Defaults.vi"("User"=w149) -> ("Params"=w155:T14, "Threshold Estimation"=w143:T13, "settings"=w150:path)  [unwired: 12 in]
            n53 = local write "Tab Control"(enum32{"Stimulus", "Masker"}."Stimulus" ("Tab Control")) -> ()
            n54 = call "FileIO-File or Folder Exists.vi"("path"=w150) -> ("Exists?"=w151:bool, "dup path"=w154:path)  [unwired: 7 in, 2 out]
            n55 = case shown="True" w151 {
              tunnel: w154 -> [_ w158]
              tunnel: [path "--- defaults ---" ("selected") w158] -> w153
              frame False {
                n56 = property on="redisplay" class="Bool (strict)"("Val(Sgnl)"=TRUE ("Value (Signaling)")) -> ()  [unwired: 2 in, 2 out]
              }
              frame True {
                n57 = property on="settings" class="Path"("Val(Sgnl)"=w158) -> ()  [unwired: 2 in, 2 out]
              }
            }
            n58 = control-ref of="Presets"() -> (w152:refnum<vi>)
            n59 = call "FileIO-Update Parameter File Presets.vi"("Presets"=w152, "folder"=w148, "selected"=w153) -> ()  [unwired: 13 in]
            n60 = property on="I-O" class="XYGraph (strict)"("Value"=w146, "Active Cursor"=u32 0, "Cursor.Visible"=FALSE) -> ()  [unwired: 2 in, 2 out]
            n61 = local write "Neural"(w146) -> ()
            n62 = local write "CM"(w146) -> ()
            n63 = local write "Wave 1"(w146) -> ()
          }
        }
        n64 = property on="Start" class="Bool"("Visible"=w137) -> ()  [unwired: 2 in, 2 out]
        n65 = property on="Exit" class="Bool"("Visible"=w137) -> ()  [unwired: 2 in, 2 out]
        n66 = vi-ref "ABR3-Averager.vi"() -> (w139:refnum<vi>)
        n67 = invoke on="Sub Panel" class="SubPanel" method="Insert VI"("VI Ref"=w139) -> ()  [unwired: 3 in, 4 out]
        n68 = local write "DataPath"(path "" ("Datafile path")) -> ()
        "Abort" <- w136
        "Running" <- w136
      }
      event Panel Close? {
        n69 = event-data() -> ()  [unwired: 1 in, 1 out]
        n70 = property on="exit signal" class="Bool (strict)"("Val(Sgnl)"=TRUE ("Value (Signaling)")) -> ()  [unwired: 2 in, 2 out]
        n71 = event-data("Discard?"=TRUE) -> ()  [unwired: 1 in, 1 out]
      }
      event "Exit", "exit signal": Value Change {
        n72 = event-data() -> ()  [unwired: 1 in, 1 out]
        n73 = call "CFTS-Is Advanced User.vi"("Experimenter"=w168) -> ("Advanced user"=w175:bool)
        n74 = Concatenate Strings(":" ("string"), w168) -> (w173:string)
        n75 = Select(t=w173, s=w175, f="") -> (s? t:f=w170:string)
        n76 = Concatenate Strings("ABR3" ("Section Name (Name of \"Type of Anything\")"), w170) -> (w169:string)
        n77 = local read "settings"() -> (w177:path)
        n78 = call "Default Config File Path.vi"() -> ("Default config file name"=w176:path)
        n79 = call "Write Anything.vi"("Section Name (Name of \"Anything\")"=w169, "Anything"=w177, "Path (dialog)"=w176) -> ("Error Out"=w165:errorcluster, "Path out"=w166:path)  [unwired: 7 in]
        n80 = call "Write Anything.vi"("Error In"=w165, "Section Name (Name of \"Anything\")"="ABR Threshold" ("Section Name (Name of \"Anything\")"), "Anything"=w164, "Path (dialog)"=w166) -> ()  [unwired: 6 in, 2 out]
      }
      event Key Down {
        n81 = event-data() -> ("ScanCode"=w186:i16, "PlatMods"=w185:T50)  [unwired: 1 in]
        n82 = Unbundle By Name(w185) -> ("Shift"=w189:bool, "Ctrl"=w188:bool)
        n83 = Equal?(x=i16 37 ("y"), y=w186) -> (x = y?=w190:bool)
        n84 = Compound Arithmetic op=AND(w190, w189, w188) -> (w187:bool)
        n85 = Stop(stop? (T)=w187) -> ()
      }
      event Menu Selection (User) {
        n86 = event-data() -> ("ItemTag"=w197:string)  [unwired: 1 in]
        n87 = Unbundle By Name(w199) -> ("Data Folder"=w198:path)
        n88 = case shown="\"mmFileOpen\"" w197 {
          selector: w197 -> [_ _ w214 _ _ _ _]
          tunnel: w198 -> [_ _ _ w231 _ _ _]
          tunnel: w196 -> [_ _ w213 _ _ _ _]
          tunnel: w195 -> [w202 w204 w207 w226 w261 w264 w271]
          tunnel: [w202 w204 w207 w226 w261 w264 w270] -> w194
          tunnel: w193 -> [w201 w203 w206 w224 w260 w263 w268]
          tunnel: [w201 w203 w206 w224 w260 w263 w267] -> w192
          frame "False", Default {
          }
          frame "mmFileLoad" {
            n89 = property on="load params" class="Bool (strict)"("Val(Sgnl)"=TRUE) -> ()  [unwired: 2 in, 2 out]
          }
          frame "mmFileSave", "mmFileSaveAs" {
            n90 = local read "settings"() -> (w212:path)
            n91 = Equal?(x=w214, y="mmFileSaveAs") -> (x = y?=w218:bool)
            n92 = call "FileIO-File or Folder Exists.vi"("path"=w212) -> ("Exists?"=w209:bool, "dup path"=w211:path)  [unwired: 7 in, 2 out]
            n93 = Not(x=w209) -> (.not. x?=w208:bool)
            n94 = Or(x=w208, y=w218) -> (x .or. y?=w210:bool)
            n95 = call "FileIO-Write Parameters.vi"("Parameter File"=w211, "Default Folder"=w213, "Parameters"=w207, "Prompt? (T)"=w210) -> ("selected path"=w217:path, "saved"=w216:bool, "error out"=w215:errorcluster)  [unwired: 9 in]
            n96 = case shown="True" w216 {
              tunnel: w217 -> [_ w220]
              tunnel: w215 -> [_ _]
              tunnel: w213 -> [_ w221]
              frame False {
              }
              frame True {
                n97 = control-ref of="Presets"() -> (w222:refnum<vi>)
                n98 = call "FileIO-Update Parameter File Presets.vi"("Presets"=w222, "folder"=w221, "selected"=w220) -> ()  [unwired: 13 in]
                n99 = local write "settings"(w220) -> ()
                n100 = One Button Dialog(message="Parameters saved.") -> ()  [unwired: 1 in, 1 out]
              }
            }
          }
          frame "mmFileOpen" {
            n101 = call "FileIO-Open Dialog (multiple).vi"("Default Folder"=w231, "pattern (all files)"="*") -> ("error out"=w230:errorcluster, "cancelled"=w225:bool, "Paths"=w229:path[])  [unwired: 7 in]
            n102 = Index Array(array=w229) -> (element=w228:path)  [unwired: 1 in]
            n103 = case shown="False" w225 {
              tunnel: w230 -> [w250 _]
              tunnel: w228 -> [w249 _]
              tunnel: w224 -> [w234 _]
              frame False {
                n104 = call "ABR3-Read Data.vi"("Path"=w249, "error in (no error)"=w250) -> ("Analysis"=w239:T9, "error out"=w241:errorcluster)  [unwired: 8 in, 4 out]
                n105 = Unbundle By Name(w239) -> ("threshold"=w238:dbl)
                n106 = local read "Normalize traces"() -> (w246:T12)
                n107 = control-ref of="I-O"() -> (w247:refnum<vi>)
                n108 = control-ref of="Neural"() -> (w243:refnum<vi>)
                n109 = control-ref of="CM"() -> (w242:refnum<vi>)
                n110 = Not A Number/Path/Refnum?(number/path/refnum=w238) -> (NaN/Path/Refnum?=w237:bool)
                n111 = case shown="True" w237 {
                  tunnel: w241 -> [w253 w259]
                  tunnel: [w253 w258] -> w240
                  tunnel: w239 -> [w254 w257]
                  tunnel: [w254 w256] -> w233
                  tunnel: w234 -> [_ w255]
                  frame False {
                  }
                  frame True {
                    n112 = call "ABR3-Estimate Threshold (wrapper).vi"("Threshold Estimation"=w255, "error in (no error)"=w259, "Analysis (in)"=w257) -> ("Analysis (out)"=w256:T9, "error out"=w258:errorcluster)  [unwired: 10 in, 1 out]
                  }
                }
                n113 = call "ABR3-Plot Metrics.vi"("Analysis"=w233, "error in (no error)"=w240, "I-O"=w247) -> ("error out"=w248:errorcluster)  [unwired: 12 in]
                n114 = Unbundle By Name(w233) -> ("threshold"=w236:dbl)
                n115 = Unbundle By Name(w233) -> ("ThrResult"=w232:T10)
                n116 = call "ABR3-Plot Traces.vi"("Analysis"=w233, "Normalize individual?"=w246, "error in (no error)"=w248, "Neural Ref"=w243, "CM Ref"=w242) -> ("error out"=w245:errorcluster)  [unwired: 10 in]
                n117 = call "ABR3-Threshold To String.vi"("Threshold"=w236) -> ("String"=w235:string)
                n118 = property on="Analysis" class="Clust (strict)"(error in=w245, "Val(Sgnl)"=w233) -> (error out=w244:errorcluster)  [unwired: 1 in, 1 out]
                n119 = case shown="\"Power (noisy)\", \"Suprathreshold\"" w232 {
                  selector: w232 -> [_ w252]
                  frame "None", Default {
                  }
                  frame "Power (noisy)", "Suprathreshold" {
                    n120 = control-ref of="This VI"() -> (w251:refnum<vi>)
                    n121 = call "ABR3-Threshold Warning Dialog.vi"("Result"=w252, "Parent VI"=w251) -> ()  [unwired: 14 in]
                  }
                }
                n122 = local write "Thr"(w235) -> ()
                n123 = call "Error Handler.vi"("error in (no error)"=w244) -> ()  [unwired: 13 in, 2 out]
              }
              frame True {
              }
            }
          }
          frame "mmFileResume" {
            n124 = property on="resume signal" class="Bool (strict)"("Val(Sgnl)"=TRUE ("Value (Signaling)")) -> ()  [unwired: 2 in, 2 out]
          }
          frame "mmFileExit" {
            n125 = property on="exit signal" class="Bool (strict)"("Val(Sgnl)"=TRUE ("Value (Signaling)")) -> ()  [unwired: 2 in, 2 out]
          }
          frame "mmEditOptions" {
            n126 = Unbundle By Name(w271) -> ("Hidden"=w269:T20)
            n127 = control-ref of="This VI"() -> (w266:refnum<vi>)
            n128 = call "ABR3-Options Dialog.vi"("Hidden"=w269, "Parent VI"=w266, "Threshold Estimation In"=w268) -> ("Cluster out"=w272:T20, "Threshold Estimation Out"=w267:T13)  [unwired: 10 in, 1 out]
            n129 = Bundle By Name(cluster=w271, "Hidden"=w272) -> (w270:T14)
          }
        }
      }
      event "I-O": Shortcut Menu Activation? {
        n130 = event-data() -> ()  [unwired: 1 in, 1 out]
        n131 = local read "Analysis"() -> (w276:T9)
        n132 = Unbundle By Name(w276) -> ("Neural"=w275:dbl[][])
        n133 = Empty Array?(array=w275) -> (empty?=w274:bool)
        n134 = event-data("Discard?"=w274) -> ()  [unwired: 1 in, 1 out]
      }
      event "I-O": Shortcut Menu Selection (User) {
        n135 = event-data() -> ()  [unwired: 1 in, 1 out]
        n136 = local read "Analysis"() -> (w280:T9)
        n137 = call "ABR3-Estimate Threshold (wrapper).vi"("Analysis (in)"=w280) -> ("Work"=w281:T51)  [unwired: 12 in, 2 out]
        n138 = call "ABR3-Show Threshold Estimation Work.vi"("work"=w281) -> ()  [unwired: 15 in]
      }
      event "redisplay": Value Change {
        n139 = event-data() -> ()  [unwired: 1 in, 1 out]
        n140 = Unbundle By Name(w294) -> ("CAP or ABR"=w293:enum16{"CAP", "ABR"}, "Stimulus"=w292:T15, "Masker"=w286:T4, "Sequence"=w291:T17, "Controls"=w290:T18, "Response"=w289:T19, "Masker.Use masker"=w288:bool, "Stimulus.Waveform"=w287:T16, "Stimulus.Chirp.Type"=w285:enum16{"AN latency-corrected", "Arbitrary"})
        n141 = local write "CAP or ABR"(w293) -> ()
        n142 = local write "Stimulus"(w292) -> ()
        n143 = local write "Sequence"(w291) -> ()
        n144 = local write "Controls"(w290) -> ()
        n145 = local write "Response"(w289) -> ()
        n146 = property on="Use masker" class="Bool (strict)"("Val(Sgnl)"=w288) -> ()  [unwired: 2 in, 2 out]
        n147 = property on="Waveform" class="Enum (strict)"("Val(Sgnl)"=w287) -> ()  [unwired: 2 in, 2 out]
        n148 = property on="Type" class="Enum (strict)"("Val(Sgnl)"=w285) -> ()  [unwired: 2 in, 2 out]
        n149 = property on="Masker" class="Clust (strict)"("Val(Sgnl)"=w286) -> ()  [unwired: 2 in, 2 out]
      }
      event "Presets": Value Change {
        n150 = event-data() -> ("CtlRef"=w299:refnum<vi>)  [unwired: 1 in]
        n151 = call "FileIO-Get Preset Parameter File.vi"("Presets"=w299, "folder"=w300) -> ("selected"=w301:path)  [unwired: 12 in, 1 out]
        n152 = Path To String(path=w301) -> (string=w302:string)
        n153 = case shown="\"--- defaults ---\"" w302 {
          tunnel: w298 -> [w305 _]
          tunnel: [w305 w306] -> w297
          tunnel: w301 -> [w304 _]
          frame "False", Default {
            n154 = property on="settings" class="Path"("Val(Sgnl)"=w304) -> ()  [unwired: 2 in, 2 out]
          }
          frame "--- defaults ---" {
            n155 = property on="redisplay" class="Bool (strict)"("Val(Sgnl)"=TRUE ("Value (Signaling)")) -> ()  [unwired: 2 in, 2 out]
            n156 = call "ABR3-Restore Defaults.vi"() -> ("Params"=w306:T14)  [unwired: 13 in, 2 out]
          }
        }
      }
      event "Presets": Shortcut Menu Activation? {
        n157 = event-data() -> ("CtlRef"=w312:refnum<vi>)  [unwired: 1 in]
        n158 = property class="Ring (strict)"(reference=w312) -> ("RingText.Text"=w311:string)  [unwired: 1 in, 2 out]
        n159 = Equal?(x=w311, y="--- defaults ---") -> (x = y?=w309:bool)
        n160 = event-data("Discard?"=w309) -> ()  [unwired: 1 in, 1 out]
      }
      event "Presets": Shortcut Menu Selection (User) {
        n161 = event-data() -> ("CtlRef"=w316:refnum<vi>, "ItemTag"=w319:string)  [unwired: 1 in]
        n162 = case shown="\"pmDelete\"" w319 {
          tunnel: w318 -> [_ _]
          tunnel: w317 -> [_ w322]
          tunnel: w316 -> [_ w323]
          frame "False", Default {
          }
          frame "pmDelete" {
            n163 = call "FileIO-Get Preset Parameter File.vi"("Presets"=w323, "folder"=w322) -> ("Name"=w326:string, "selected"=w324:path)  [unwired: 12 in]
            n164 = Format Into String(format string="Delete '%s'?" ("message"), w326) -> (resulting string=w329:string)  [unwired: 2 in, 1 out]
            n165 = local read "Presets"() -> (w321:u16)
            n166 = Two Button Dialog(message=w329, 1:"No" ("F button name (\"Cancel\")"), 2:"Yes" ("T button name (\"OK\")")) -> (T button?=w325:bool)
            n167 = case shown="True" w325 {
              tunnel: w324 -> [_ w338]
              tunnel: w323 -> [_ w333]
              tunnel: w322 -> [_ w335]
              tunnel: w321 -> [_ w331]
              frame False {
              }
              frame True {
                n168 = Delete(path (use dialog)=w338) -> (error out=w334:errorcluster)  [unwired: 4 in, 2 out]
                n169 = call "FileIO-List Parameter Files.vi"("folder"=w335, "error in (no error)"=w334) -> ("Parameter file names"=w337:string[])  [unwired: 13 in]
                n170 = Build Array (concatenate)(w337, "--- defaults ---") -> (w332:string[])
                n171 = property class="Ring (strict)"(reference=w333, "Strings []"=w332, "Val(Sgnl)"=w331) -> ()  [unwired: 1 in, 2 out]
              }
            }
          }
        }
      }
      event "settings", "load params": Value Change {
        n172 = event-data() -> ("CtlRef"=w342:refnum<vi>)  [unwired: 1 in]
        n173 = control-ref of="load params"() -> (w344:refnum<vi>)
        n174 = local read "settings"() -> (w346:path)
        n175 = Equal?(x=w342, y=w344) -> (x = y?=w345:bool)
        n176 = call "FileIO-Read Parameters.vi"("Settings file"=w346, "Type of Parameters"=w343, "Default Folder"=w341, "Prompt?"=w345) -> ("Path out"=w349:path, "Anything"=w348:variant, "Read?"=w347:bool)  [unwired: 7 in, 2 out]
        n177 = case shown="True" w347 {
          tunnel: w348 -> [_ w359]
          tunnel: w343 -> [w354 w358]
          tunnel: [w354 w357] -> w340
          tunnel: w349 -> [w353 w355]
          tunnel: [w353 w355] -> w351
          frame False {
          }
          frame True {
            n178 = Variant To Data(type=w358, Variant=w359) -> (data=w357:T14)  [unwired: 1 in, 1 out]
            n179 = property on="redisplay" class="Bool (strict)"("Val(Sgnl)"=TRUE ("Value (Signaling)")) -> ()  [unwired: 2 in, 2 out]
            "settings" <- w355
          }
        }
        n180 = control-ref of="Presets"() -> (w350:refnum<vi>)
        n181 = call "FileIO-Update Parameter File Presets.vi"("Presets"=w350, "folder"=w341, "selected"=w351) -> ()  [unwired: 13 in]
      }
      event "CAP or ABR": Value Change {
        n182 = event-data() -> ()  [unwired: 1 in, 1 out]
        n183 = Bundle By Name(cluster=w363, "CAP or ABR"="CAP or ABR") -> (w362:T14)
      }
      event "Stimulus": Value Change {
        n184 = event-data() -> ("NewVal"=w366:T3)  [unwired: 1 in]
        n185 = Bundle By Name(cluster=w368, "Stimulus"=w366) -> (w367:T14)
      }
      event "Stimulus.Waveform": Value Change {
        n186 = event-data() -> ("NewVal"=w377:T52)  [unwired: 1 in]
        n187 = case shown="\"NOISE\"" w377 {
          tunnel: [FALSE FALSE w390 FALSE FALSE] -> w376
          tunnel: [w381 w385 w390 FALSE FALSE] -> w375
          tunnel: [w381 w385 FALSE TRUE FALSE] -> w374
          tunnel: [FALSE TRUE FALSE FALSE FALSE] -> w372
          tunnel: [FALSE FALSE FALSE FALSE TRUE] -> w371
          frame "CLICK", Default {
            w381 = FALSE
          }
          frame "CHIRP" {
            w385 = FALSE
          }
          frame "FILE" {
            w390 = TRUE
          }
          frame "TONE PIP" {
          }
          frame "NOISE" {
          }
        }
        n188 = property on="Filenames" class="Str"("Visible"=w376) -> ()  [unwired: 2 in, 2 out]
        n189 = property on="Frequency (kHz)" class="Str"("Visible"=w374) -> ()  [unwired: 2 in, 2 out]
        n190 = property on="File browse" class="Bool"("Visible"=w375) -> ()  [unwired: 2 in, 2 out]
        n191 = property on="Noise" class="Clust (strict)"("Visible"=w371) -> ()  [unwired: 2 in, 2 out]
        n192 = property on="Chirp" class="Clust (strict)"("Visible"=w372) -> ()  [unwired: 2 in, 2 out]
      }
      event "Stimulus.Chirp.Type": Value Change {
        n193 = event-data() -> ("NewVal"=w404:enum16{"AN latency-corrected", "Arbitrary"})  [unwired: 1 in]
        n194 = Equal?(x=w404, y=enum16{"AN latency-corrected", "Arbitrary"}."Arbitrary") -> (x = y?=w402:bool)
        n195 = property on="Fmax (kHz)" class="DigNum (strict)"("Visible"=w402) -> ()  [unwired: 2 in, 2 out]
        n196 = property on="Precompensate" class="Bool (strict)"("Visible"=w402) -> ()  [unwired: 2 in, 2 out]
        n197 = property on="Fmin (kHz)" class="DigNum (strict)"("Visible"=w402) -> ()  [unwired: 2 in, 2 out]
        n198 = property on="Duration (ms)" class="DigNum (strict)"("Visible"=w402) -> ()  [unwired: 2 in, 2 out]
      }
      event Value Change {
        n199 = event-data() -> ("NewVal"=w408:T4)  [unwired: 1 in]
        n200 = Bundle By Name(cluster=w410, "Masker"=w408) -> (w409:T14)
      }
      event Value Change {
        n201 = event-data() -> ("NewVal"=w414:bool)  [unwired: 1 in]
        n202 = property on="Masker state" class="Bool (strict)"("Value"=w414) -> ()  [unwired: 2 in, 2 out]
        n203 = Select(t=T49."Enabled" ("Disabled"), s=w414, f=T49."Disabled and Grayed Out" ("Disabled")) -> (s? t:f=w415:T49)
        n204 = property on="Filter" class="Advanced Filter XCtl (strict)"("DisabledEnum"=w415) -> (error out=w420:errorcluster)  [unwired: 2 in, 1 out]
        n205 = property on="Level" class="Level XCtl (strict)"(error in=w420, "DisabledEnum"=w415) -> (error out=w418:errorcluster)  [unwired: 1 in, 1 out]
        n206 = property on="Audiogram Comp" class="Bool (strict)"(error in=w418, "DisabledEnum"=w415) -> (error out=w417:errorcluster)  [unwired: 1 in, 1 out]
        n207 = property on="Audiogram File" class="Path"(error in=w417, "DisabledEnum"=w415) -> (error out=w416:errorcluster)  [unwired: 1 in, 1 out]
        n208 = property on="InvFilt" class="Bool (strict)"(error in=w416, "DisabledEnum"=w415) -> ()  [unwired: 1 in, 2 out]
      }
      event "Sequence": Value Change {
        n209 = event-data() -> ("NewVal"=w424:T7)  [unwired: 1 in]
        n210 = Bundle By Name(cluster=w426, "Sequence"=w424) -> (w425:T14)
      }
      event "Controls": Value Change {
        n211 = event-data() -> ("NewVal"=w429:T6)  [unwired: 1 in]
        n212 = Bundle By Name(cluster=w431, "Controls"=w429) -> (w430:T14)
      }
      event "Response": Value Change {
        n213 = event-data() -> ("NewVal"=w434:T8)  [unwired: 1 in]
        n214 = Bundle By Name(cluster=w436, "Response"=w434) -> (w435:T14)
      }
      event "Start": Value Change {
        w445 = FALSE ("ABI Abort")
        n215 = event-data() -> ()  [unwired: 1 in, 1 out]
        n216 = Bundle("Params"=w440, "Threshold Estimation Out"=w439) -> (w438:T53)  [unwired: 1 in]
        n217 = Send Notification(notification=w438, notifier=w441) -> ()  [unwired: 1 in, 2 out]
        n218 = Unbundle By Name(w440) -> ("Stimulus.Waveform"=w442:T16)
        n219 = local write "Abort"(w445) -> ()
        n220 = property on="Exit" class="Bool"("Visible"=w445) -> ()  [unwired: 2 in, 2 out]
        n221 = property on="Start" class="Bool"("Visible"=w445) -> ()  [unwired: 2 in, 2 out]
        n222 = local write "Stop"(w445) -> ()
        n223 = case shown="\"FILE\"" w442 {
          frame "CLICK" {
            n224 = property on="kHz" class="DigNum (strict)"("Visible"=FALSE) -> ()  [unwired: 2 in, 2 out]
          }
          frame "FILE" {
            n225 = property on="kHz" class="DigNum (strict)"("Visible"=TRUE, "Caption.Text"="File #") -> ()  [unwired: 2 in, 2 out]
          }
          frame "TONE PIP", Default {
            n226 = property on="kHz" class="DigNum (strict)"("Visible"=TRUE, "Caption.Text"="kHz") -> ()  [unwired: 2 in, 2 out]
          }
        }
        n227 = local write "Running"(TRUE ("Running")) -> ()
        n228 = local write "NOTES"("" ("NOTES")) -> ()
      }
      event "resume signal": Value Change {
        n229 = event-data() -> ()  [unwired: 1 in, 1 out]
        n230 = local read "Analysis"() -> (w456:T9)
        n231 = Unbundle By Name(w456) -> ("Aborted"=w455:bool)
        n232 = case shown="True" w455 {
          tunnel: w454 -> [_ w461]
          tunnel: w453 -> [_ w460]
          tunnel: w452 -> [_ w459]
          frame False {
            n233 = One Button Dialog(message="The previous measurement cannot be resumed.") -> ()  [unwired: 1 in, 1 out]
          }
          frame True {
            n234 = Two Button Dialog(message="Are you sure you want to resume the previous measurement?", 1:"No" ("F button name (\"Cancel\")"), 2:"Yes" ("T button name (\"OK\")")) -> (T button?=w462:bool)
            n235 = case shown="True" w462 {
              tunnel: w461 -> [_ w469]
              tunnel: w460 -> [_ w468]
              tunnel: w459 -> [_ w466]
              frame False {
              }
              frame True {
                n236 = Bundle("Params"=w468, "Threshold Estimation Out"=w466) -> (w467:T53)  [unwired: 1 in]
                n237 = Send Notification(notification=w467, notifier=w469) -> ()  [unwired: 1 in, 2 out]
              }
            }
          }
        }
      }
      event "Stop": Value Change {
        n238 = event-data() -> ()  [unwired: 1 in, 1 out]
        n239 = local write "Abort"(TRUE ("Stopping")) -> ()
      }
      event "finished": Value Change {
        w485 = FALSE ("Running")
        w484 = TRUE
        n240 = event-data() -> ()  [unwired: 1 in, 1 out]
        n241 = local read "Analysis"() -> (w475:T9)
        n242 = local read "Normalize traces"() -> (w479:T12)
        n243 = control-ref of="I-O"() -> (w478:refnum<vi>)
        n244 = control-ref of="Neural"() -> (w480:refnum<vi>)
        n245 = control-ref of="CM"() -> (w481:refnum<vi>)
        n246 = call "ABR3-Plot Metrics.vi"("Analysis"=w475, "I-O"=w478) -> ("error out"=w477:errorcluster)  [unwired: 13 in]
        n247 = Unbundle By Name(w475) -> ("ThrResult"=w474:T10)
        n248 = call "ABR3-Plot Traces.vi"("Analysis"=w475, "Normalize individual?"=w479, "error in (no error)"=w477, "Neural Ref"=w480, "CM Ref"=w481) -> ()  [unwired: 10 in, 1 out]
        n249 = case shown="\"Power (noisy)\", \"Suprathreshold\"" w474 {
          selector: w474 -> [_ w488]
          frame "None", Default {
          }
          frame "Power (noisy)", "Suprathreshold" {
            n250 = control-ref of="This VI"() -> (w487:refnum<vi>)
            n251 = call "ABR3-Threshold Warning Dialog.vi"("Result"=w488, "Parent VI"=w487) -> ()  [unwired: 14 in]
          }
        }
        n252 = local write "Running"(w485) -> ()
        n253 = local write "Stop"(w485) -> ()
        n254 = call "Beeper.vi"() -> ()  [unwired: 5 in, 1 out]
        n255 = property on="Exit" class="Bool"("Visible"=w484) -> ()  [unwired: 2 in, 2 out]
        n256 = property on="Start" class="Bool"("Visible"=w484) -> ()  [unwired: 2 in, 2 out]
        n257 = call "Error Handler.vi"("error in (no error)"="finished") -> ()  [unwired: 13 in, 2 out]
      }
      event "File browse": Value Change {
        w500 = T54 2 items=["User Home"=0, "User Desktop"=1, "User Documents"=2, "User Application Data"=3, "User Preferences"=4, "User Temporary"=5, "Public Documents"=6, "Public Application Data"=7, "Public Preferences"=8, "Public Cache"=13, "System Core Libraries"=9, "System Installed Libraries"=10, "Application Files"=11, "Boot Volume Root"=12] ("system directory type")
        n258 = event-data() -> ()  [unwired: 1 in, 1 out]
        n259 = local read "Stimulus"() -> (w497:T3)
        n260 = Unbundle By Name(w497) -> ("Folder"=w501:path)
        n261 = call <vilib>:"Get System Directory.vi"("system directory type"=w500) -> ("system directory"=w499:path)  [unwired: 10 in]
        n262 = call "FileIO-Open Dialog (multiple).vi"("Default Folder"=w499, "pattern (all files)"="*.wav", "Start path"=w501) -> ("Paths"=w498:path[])  [unwired: 6 in, 2 out]
        n263 = for {
          tunnel: w498 -> [w507] mode=indexing
          shift-right: [w509] -> w496
          shift-left: "" -> [w508]
          tunnel: [w505] -> w495
          n264 = Strip Path(path=w507) -> (stripped path=w505:path, name=w506:string)
          n265 = Concatenate Strings(w508, w506, "\r") -> (w509:string)
        }
        n266 = Bundle By Name(cluster=w497, "Folder"=w495, "Filenames"=w496) -> (w490:T3)
        n267 = property on="Stimulus" class="Clust (strict)"("Value"=w490) -> (error out=w493:errorcluster)  [unwired: 2 in, 1 out]
        n268 = Bundle By Name(cluster=w492, "Stimulus"=w490) -> (w491:T14)
      }
      event Value Change {
        n269 = event-data() -> ("NewVal"=w514:T12)  [unwired: 1 in]
        n270 = case shown="False" FALSE {
          tunnel: w514 -> [w518 _]
          frame False {
            n271 = local read "Analysis"() -> (w517:T9)
            n272 = control-ref of="Neural"() -> (w516:refnum<vi>)
            n273 = control-ref of="CM"() -> (w515:refnum<vi>)
            n274 = call "ABR3-Plot Traces.vi"("Analysis"=w517, "Normalize individual?"=w518, "Neural Ref"=w516, "CM Ref"=w515) -> ()  [unwired: 11 in, 1 out]
          }
          frame True {
          }
        }
      }
      event "NOTES": Value Change {
        n275 = event-data() -> ("NewVal"=w523:string)  [unwired: 1 in]
        n276 = local read "Running"() -> (w529:bool)
        n277 = local read "DataPath"() -> (w524:path)
        n278 = Not(x=w529) -> (.not. x?=w527:bool)
        n279 = Empty String/Path?(string/path=w524) -> (empty?=w528:bool)
        n280 = Not(x=w528) -> (.not. x?=w526:bool)
        n281 = And(x=w526, y=w527) -> (x .and. y?=w525:bool)
        n282 = case shown="True" w525 {
          tunnel: w524 -> [_ w533]
          tunnel: w523 -> [_ w532]
          tunnel: "Add notes to data file?" ("message") -> [_ w531]
          frame False {
          }
          frame True {
            n283 = Two Button Dialog(message=w531) -> (T button?=w530:bool)  [unwired: 2 in]
            n284 = case shown="True" w530 {
              tunnel: w533 -> [_ w535]
              tunnel: w532 -> [_ w534]
              frame False {
              }
              frame True {
                n285 = call "ABR-Insert Notes.vi"("path"=w535, "Notes"=w534) -> ()  [unwired: 12 in, 2 out]
              }
            }
          }
        }
      }
      event Value Change; "Neural": Cursor Release {
        n286 = event-data() -> ()  [unwired: 1 in, 1 out]
        n287 = local read "Analysis"() -> (w544:T9)
        n288 = control-ref of="Wave 1"() -> (w539:refnum<vi>)
        n289 = property on="Neural" class="XYGraph (strict)"() -> ("Cursor.Cursor X"=w537:dbl)  [unwired: 2 in, 2 out]
        n290 = call "ABR3-Analyze With User Window.vi"("Analysis"=w544, "Tmax (ms)"=w537) -> ("Analysis Out"=w541:T9, "error out"=w543:errorcluster)  [unwired: 12 in]
        "Analysis" <- w541
        n291 = call "ABR3-Plot Metrics.vi"("Analysis"=w541, "Plot user metric?"=TRUE, "error in (no error)"=w543, "I-O"=w539) -> ("error out"=w542:errorcluster)  [unwired: 11 in]
        n292 = call "Error Handler.vi"("error in (no error)"=w542) -> ()  [unwired: 13 in, 2 out]
      }
    }
  }
  n293 = Release Notifier(notifier=w18) -> ()  [unwired: 2 in, 3 out]
